vi "Check Slave Name.vi"(8 "error in (no error)":errorcluster, 9 "Prepend in":bool, 11 "Item Ref in":T1 format="%.0x") -> (0 "error out":errorcluster, 1 "Prepend out":bool, 2 "Available?":bool, 3 "Item Ref out":T1 format="%.0x", 4 "Slave Name":string)   [LabVIEW 2016, in "Scan Engine Custom Device.lvlib"]
uses:
  Scan Engine Custom Device.lvlib
  <vilib>/NI Veristand/Custom Device API/Custom Device Item Ref.ctl
  <vilib>/NI Veristand/Custom Device API/Custom Device API.lvlib
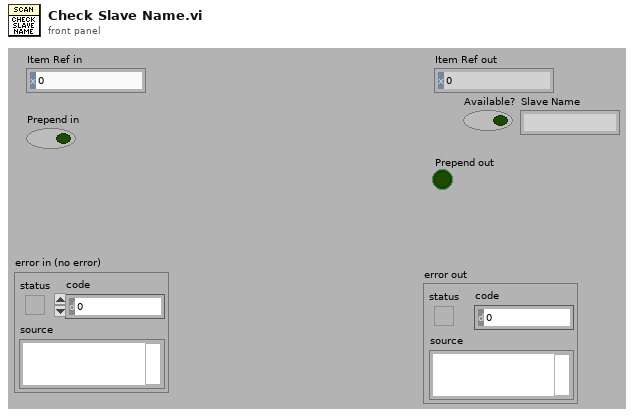
[diagram p1: front panel]
types:
  T1 = typedef "Custom Device API.lvlib/Custom Device Item Ref.ctl" = u64
  T2 = typedef "Custom Device API.lvlib/Custom Device Item Info.ctl" = cluster{"Name":string, "Is Channel":bool, "GUID":string, "Is Waveform":bool}
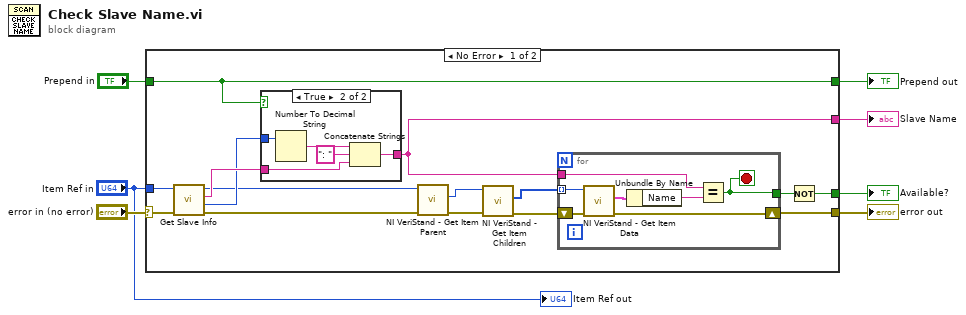
[diagram p0: block diagram]
diagram:
  n1 = case shown="No Error" "error in (no error)" {
    selector: "error in (no error)" -> [w14 w37]
    tunnel: [w19 w37] -> w6
    tunnel: "Item Ref in" -> [w15 _]
    tunnel: "Prepend in" -> [w13 w36]
    tunnel: [w13 w36] -> w4
    tunnel: [w18 _] -> w3
    tunnel: [w8 _] -> w1
    frame No Error {
      n2 = call "Get Slave Info.vi"("error in (no error)"=w14, "Item Ref in"=w15) -> ("error out"=w9:errorcluster, "Slave #"=w11:u16, "Slave Name"=w12:string, "Item Ref out"=w10:T1)  [unwired: 5 in, 1 out]
      n3 = case shown="True" w13 {
        tunnel: [w23 w28] -> w8
        tunnel: w12 -> [w23 w27]
        tunnel: w11 -> [_ w26]
        frame False {
        }
        frame True {
          n4 = Number To Decimal String(number=w26) -> (decimal integer string=w25:string)  [unwired: 1 in]
          n5 = Concatenate Strings(w25, ": " ("string"), w27) -> (w28:string)
        }
      }
      n6 = call <vilib>:"NI VeriStand - Get Item Parent.vi"("error in (no error)"=w9, "Item Ref in"=w10) -> ("error out"=w17:errorcluster, "Parent Ref"=w16:T1)  [unwired: 6 in, 2 out]
      n7 = call <vilib>:"NI VeriStand - Get Item Children.vi"("error in (no error)"=w17, "Item Ref in"=w16) -> ("error out"=w22:errorcluster, "Child Refs"=w21:T1[])  [unwired: 6 in, 2 out]
      n8 = for {
        tunnel: w21 -> [w33] mode=indexing
        shift-right: [w30] -> w19
        shift-left: w22 -> [w32]
        tunnel: [w35] -> w20
        tunnel: w8 -> [w29]
        stop <- w35 stop-if-true
        n9 = call <vilib>:"NI VeriStand - Get Item Data.vi"("error in (no error)"=w32, "Item Ref in"=w33) -> ("error out"=w30:errorcluster, "Item Info"=w34:T2)  [unwired: 8 out]
        n10 = Unbundle By Name(w34) -> ("Name"=w31:string)
        n11 = Equal?(x=w29, y=w31) -> (x = y?=w35:bool)
      }
      n12 = Not(x=w20) -> (.not. x?=w18:bool)
    }
    frame Error {
    }
  }
  "error out" <- w6
  "Available?" <- w3
  "Prepend out" <- w4
  "Slave Name" <- w1
  "Item Ref out" <- "Item Ref in"
